vi "Exp_GetSavedExperiments.vi"(8 "error in (no error)":errorcluster, 11 "LightField Automation in":refnum<class "LightField Automation.lvclass">) -> (0 "error out":errorcluster, 2 "Saved Experiments":string[](array[string]), 3 "LightField Automation out":refnum<class "LightField Automation.lvclass">)   [LabVIEW 2018, in "LightField Automation.lvclass"]
uses:
  LightField Automation.lvclass
  LightField Automation.lvclass/LightField Automation.ctl
  C:/Users/xw9/Desktop/Turbulence program/SourceDistribution/PrincetonInstruments.LightFieldViewV3.dll
  PrincetonInstruments.LightFieldViewV3.dll
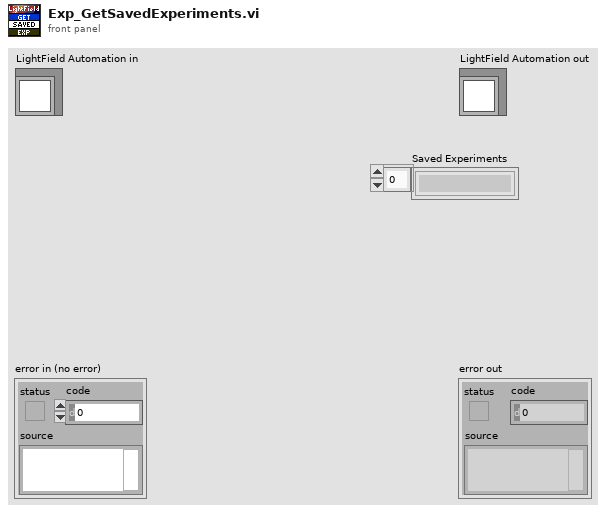
[diagram p1: front panel]
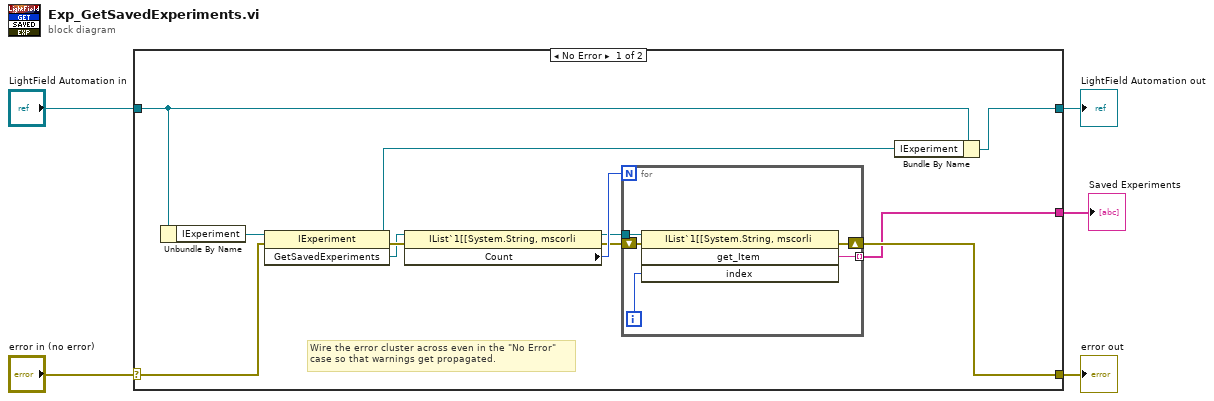
[diagram p0: block diagram]
diagram:
  n1 = case shown="No Error" "error in (no error)" {
    selector: "error in (no error)" -> [w17 w24]
    tunnel: [w9 w24] -> w4
    tunnel: [w10 w23] -> w2
    tunnel: "LightField Automation in" -> [w11 w23]
    tunnel: [w8 _] -> w1
    frame No Error {
      # "Wire the error cluster across even in the \"No Error\"\ncase so that warnings get propagated."
      n2 = Unbundle By Name(w11) -> ("IExperiment"=w7:refnum<k24>)
      n3 = invoke class="IExperiment" method="GetSavedExperiments"(reference=w7, error in=w17) -> (reference out=w6:refnum<k24>, error out=w16:errorcluster, "GetSavedExperiments"=w15:refnum<k24>)  [unwired: 1 in]
      n4 = property class="IList`1[[System.String, mscorli"(reference=w15, error in=w16) -> (reference out=w12:refnum<k24>, error out=w13:errorcluster, "Count"=w14:i32)
      n5 = for {
        N: w14 -> [_]
        shift-right: [w21] -> w9
        shift-left: w13 -> [w22]
        tunnel: w12 -> [w20]
        tunnel: [w18] -> w8 mode=indexing
        i -> [w19]
        n6 = invoke class="IList`1[[System.String, mscorli" method="get_Item"(reference=w20, error in=w22, "index"=w19) -> (error out=w21:errorcluster, "get_Item"=w18:string)  [unwired: 1 in, 2 out]
      }
      n7 = Bundle By Name(cluster=w11, "IExperiment"=w6) -> (w10:refnum<class "LightField Automation.lvclass">)
    }
    frame Error {
    }
  }
  "error out" <- w4
  "LightField Automation out" <- w2
  "Saved Experiments" <- w1
